vi "ID Query Response.vi"(8 "error in (no error)":errorcluster, 11 "VISA resource name":refnum<visa-resource-name>) -> (0 "error out":errorcluster, 2 "ID Query Response":string, 3 "VISA resource name out":refnum<visa-resource-name>)   [LabVIEW 2020, in "Rohde&Schwarz RTx Oscilloscopes.lvlib"]
doc: "This VI returns the identification string of the instrument.\n\nAttribute:\n-\n\nRemote-control command:\n*IDN?"
uses:
  Rohde&Schwarz RTx Oscilloscopes.lvlib
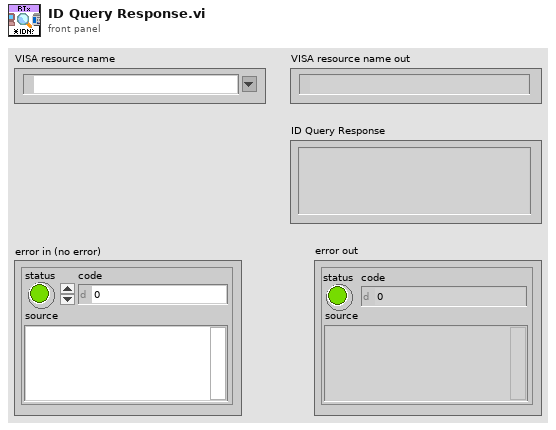
[diagram p1: front panel]
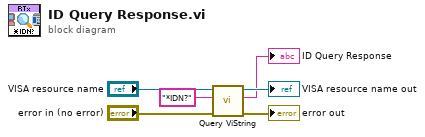
[diagram p0: block diagram]
diagram:
  n1 = call "Query ViString.vi"("error in (no error)"="error in (no error)", "Query"="*IDN?" ("Revision Query Command"), "VISA resource name"="VISA resource name") -> ("error out"=→"error out":errorcluster, "Response Value"=→"ID Query Response":string, "VISA resource name out"=→"VISA resource name out":refnum<visa-resource-name>)  [unwired: 6 in]
